vi "LLTF_Contrast_Demo.vi"() -> ()   [LabVIEW 2017]
uses:
  PE_Filter_SDK/PE_Filter_SDK.lvlib
panel:
  in  "Stop":bool
  in  "Wavelength":dbl=600.0
  out "Maximum Wavelength":dbl
  out "Minimum Wavelength":dbl
  out "Current System":string
  in  "Configuration File":path
  # "Filter Selection"
  # "Filter Information"
  # "Filter Control"
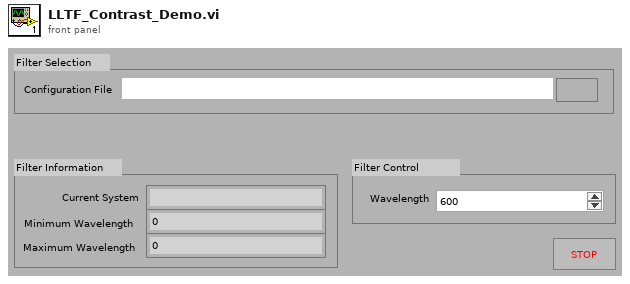
[diagram p1: front panel]
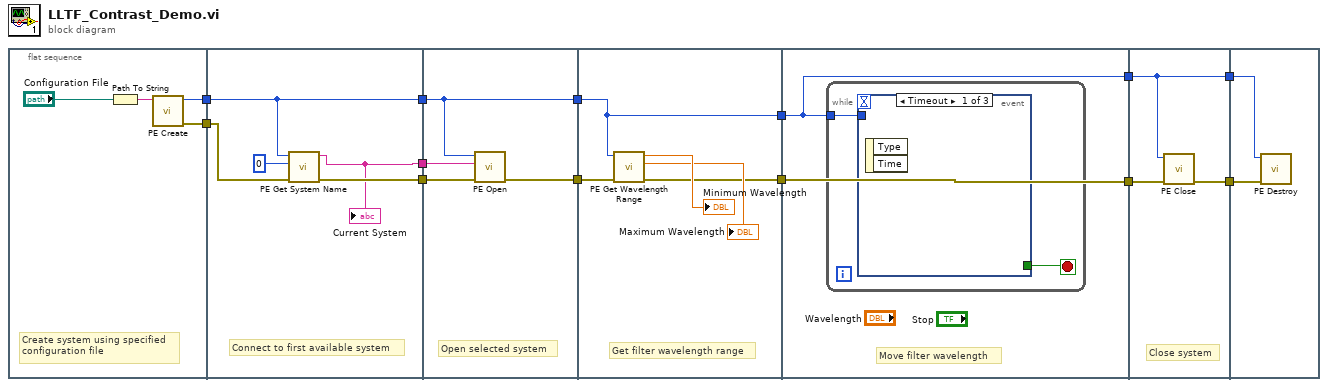
[diagram p0: block diagram]
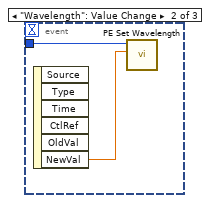
[diagram p2: hidden frame]
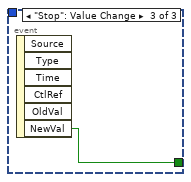
[diagram p3: hidden frame]
diagram:
  n1 = flat-sequence {
    tunnel: [w15] -> w13
    tunnel: [w14] -> w6
    tunnel: w13 -> [w21]
    tunnel: [w19] -> w9
    tunnel: [w20] -> w8
    tunnel: w6 -> [w18]
    tunnel: [w18] -> w5
    tunnel: w8 -> [w25]
    tunnel: [w26] -> w12
    tunnel: w9 -> [w24]
    tunnel: w5 -> [w23]
    tunnel: [w23] -> w4
    tunnel: w12 -> [w28]
    tunnel: [w29] -> w11
    tunnel: w4 -> [w27]
    tunnel: [w27] -> w3
    tunnel: w11 -> [w33]
    tunnel: [w33] -> w7
    tunnel: w3 -> [w32]
    tunnel: [w32] -> w2
    tunnel: [w40] -> w10
    tunnel: w7 -> [w41]
    tunnel: w2 -> [w39]
    tunnel: [w39] -> w1
    tunnel: w10 -> [w43]
    tunnel: w1 -> [w42]
    frame #0 {
      # "Create system using specified\nconfiguration file"
      n2 = Path To String(path="Configuration File") -> (string=w16:string)
      n3 = call "PE Create.vi"("conffile"=w16) -> ("error out"=w15:errorcluster, "peHandle"=w14:u32)  [unwired: 9 in]
    }
    frame #1 {
      # "Connect to first available system"
      n4 = call "PE Get System Name.vi"("error in (no error)"=w21, "index"=0, "peHandle"=w18) -> ("error out"=w20:errorcluster, "name"=w19:string)  [unwired: 6 in, 1 out]
      "Current System" <- w19
    }
    frame #2 {
      # "Open selected system"
      n5 = call "PE Open.vi"("error in (no error)"=w25, "name"=w24, "peHandle"=w23) -> ("error out"=w26:errorcluster)  [unwired: 8 in]
    }
    frame #3 {
      # "Get filter wavelength range"
      n6 = call "PE Get Wavelength Range.vi"("error in (no error)"=w28, "peHandle"=w27) -> ("error out"=w29:errorcluster, "maximum"=→"Maximum Wavelength":dbl, "minimum"=→"Minimum Wavelength":dbl)  [unwired: 7 in]
    }
    frame #4 {
      # "Move filter wavelength"
      n7 = while {
        tunnel: w32 -> [w34]
        stop <- w35 stop-if-true
        n8 = event shown="[0] Timeout" {
          selector: _ -> [_ _ _]
          dyn-events: _ -> [_ _ _]
          timeout: _ -> [_ _ _]
          tunnel: [_ _ w38] -> w35
          tunnel: w34 -> [_ w36 _]
          event Timeout {
            n9 = event-data() -> ()  [unwired: 1 in, 2 out]
          }
          event "Wavelength": Value Change {
            n10 = event-data() -> ("NewVal"=w37:dbl)  [unwired: 1 in, 5 out]
            n11 = call "PE Set Wavelength.vi"("wavelength"=w37, "peHandle"=w36) -> ()  [unwired: 9 in, 1 out]
          }
          event "Stop": Value Change {
            n12 = event-data() -> ("NewVal"=w38:bool)  [unwired: 1 in, 5 out]
          }
        }
      }
    }
    frame #5 {
      # "Close system"
      n13 = call "PE Close.vi"("error in (no error)"=w41, "peHandle"=w39) -> ("error out"=w40:errorcluster)  [unwired: 9 in]
    }
    frame #6 {
      n14 = call "PE Destroy.vi"("error in (no error)"=w43, "peHandle"=w42) -> ()  [unwired: 9 in, 1 out]
    }
  }
